vi "NI VeriStand - Get Stimulus Profile File.vi"(8 "error in (no error)":errorcluster, 11 "StimulusProfileManager in":T1) -> (0 "error out":errorcluster, 2 "File":path, 3 "StimulusProfileManager out":T1)   [LabVIEW 2020, in "NI_VS Stimulus ExecutionAPI.lvlib"]
doc: "This VI interfaces with the legacy Stimulus Profile Editor workspace tool in NI VeriStand, and is included for compatibility only. National Instruments recommends you use the current Stimulus Profile VIs to create, observe, and control NI VeriStand stimulus profiles and real-time sequences.\n\nReturns the filename of the stimulus profile file that is running on the target."
uses:
  <vilib>/NI VeriStand/Execution/Stimulus/NI_VS Stimulus ExecutionAPI.lvlib
  <vilib>/NI VeriStand/Execution/Stimulus/StimulusAPI.ctl
  NationalInstruments.VeriStand.ClientAPI
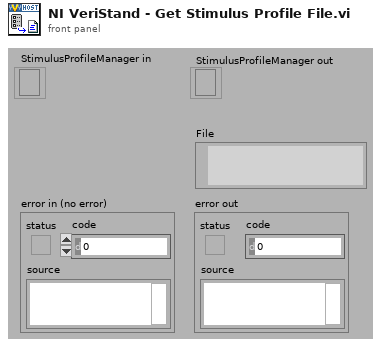
[diagram p1: front panel]
types:
  T1 = typedef "NI_VS Stimulus ExecutionAPI.lvlib/StimulusAPI.ctl" = refnum<k24>
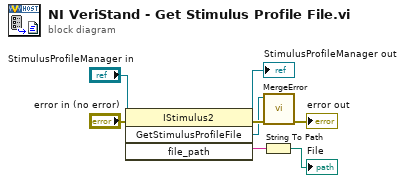
[diagram p0: block diagram]
diagram:
  n1 = invoke class="IStimulus2" method="GetStimulusProfileFile"(reference="StimulusProfileManager in", error in="error in (no error)") -> (reference out=→"StimulusProfileManager out":T1, error out=w6:errorcluster, "GetStimulusProfileFile"=w5:refnum<k24>, "file_path"=w2:string)  [unwired: 2 in]
  n2 = String To Path(string=w2) -> (path=→"File":path)
  n3 = call <vilib>:"MergeError.vi"("error in (no error)"=w6, "Error"=w5) -> ("error out"=→"error out":errorcluster)  [unwired: 9 out]
